vi "TimeTag_LSW_edits_Aug16.vi"() -> ()   [LabVIEW 2015]
doc: "This sample project is built upon the standard state machine template and shows how you could create an application that acquires, analyzes, and presents data. It includes functionality for presenting configuration dialogs, preserving settings between executions, loading and saving data, as well as exporting graph images and text files.\n\nIt is most appropriate for data that is acquired instantly as it does not allow for screen updates mid acquisition nor does it allow for continuous streaming to disk."
uses:
  <vilib>/ptbypt/NI_PtbyPt.lvlib
panel:
  out "Total Coin per sec":dbl
  out "Ch2/4 coin/sec":dbl(graph)
  out "Ch2/4 Total Coincidences":dbl
  out "Channel 2 CPS":dbl(graph)
  out "Channel 4 CPS":dbl(graph)
  out "Total Ch2 CPS":dbl
  out "Total Ch4 CPS":dbl
  in  "Averaging":dbl
  in  "Runs":dbl=100.0
  in  "Pulse TTL 2":bool
  in  "Pulse TTL 1":bool
  in  "Toggle\nTTL 2":bool
  in  "Toggle\nTTL 1":bool
  out "Total Starts":dbl
  in  "Record data":bool
  out "Initial time":dbl
  out "Elapsed time (s)":dbl
  out "FPGA_Run Status":dbl
  out "USB_Open Status":dbl
  out "Channel 4 Total\nCounts":dbl
  out "Channel 3 Total\nCounts":dbl
  out "Channel 2 Total\nCounts":dbl
  out "Channel 1 Total\nCounts":dbl
  in  "File Name":string="C:\\FPGA\\test.txt"
  out "?":dbl
  out "?":dbl
  out "?":dbl
  out "?":dbl
  out "stats":i64[](array[numeric])
  in  "Stop":bool
  out "Channel 4 CPS":dbl(knob) scale=0.0..2000000.0
  out "Channel 3 CPS":dbl(knob) scale=0.0..600.0
  out "Channel 2 CPS":dbl(knob) scale=0.0..700.0
  out "Channel 1 CPS":dbl(knob) scale=0.0..600.0
  # "Starts"
  # "Channel 1"
  # "Channel 2"
  # "Channel 3"
  # "Channel 4"
  # "Coincidence Channels 1 & 2"
  # "Coincidence Channels 1 & 3"
  # "Coincidence Channels 1 & 4"
  # "Coincidence Channels 2 & 3"
  # "Coincidence Channels 2 & 4"
  # "Coincidence Channels 3 & 4"
  # "Coincidence Channels 1 & 2 & 3"
  # "Coincidence Channels 1 & 2 & 4"
  # "Coincidence Channels 1 & 3 & 4"
  # "Coincidence Channels 2 & 3 & 4"
  # "Coincidence Channels 1 & 2 & 3 & 4"
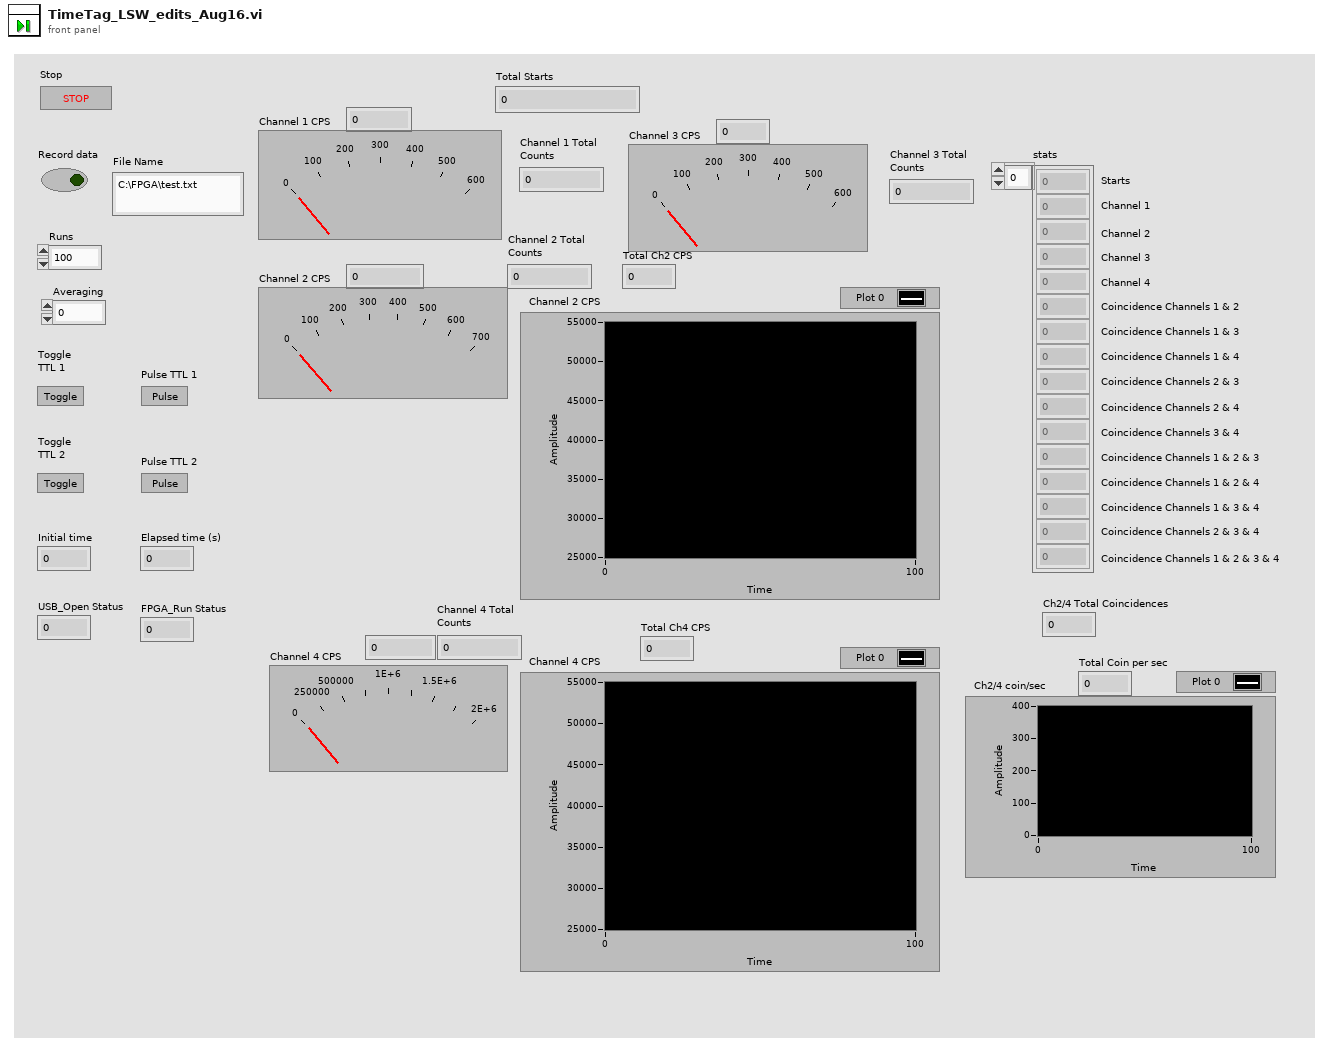
[diagram p1: front panel]
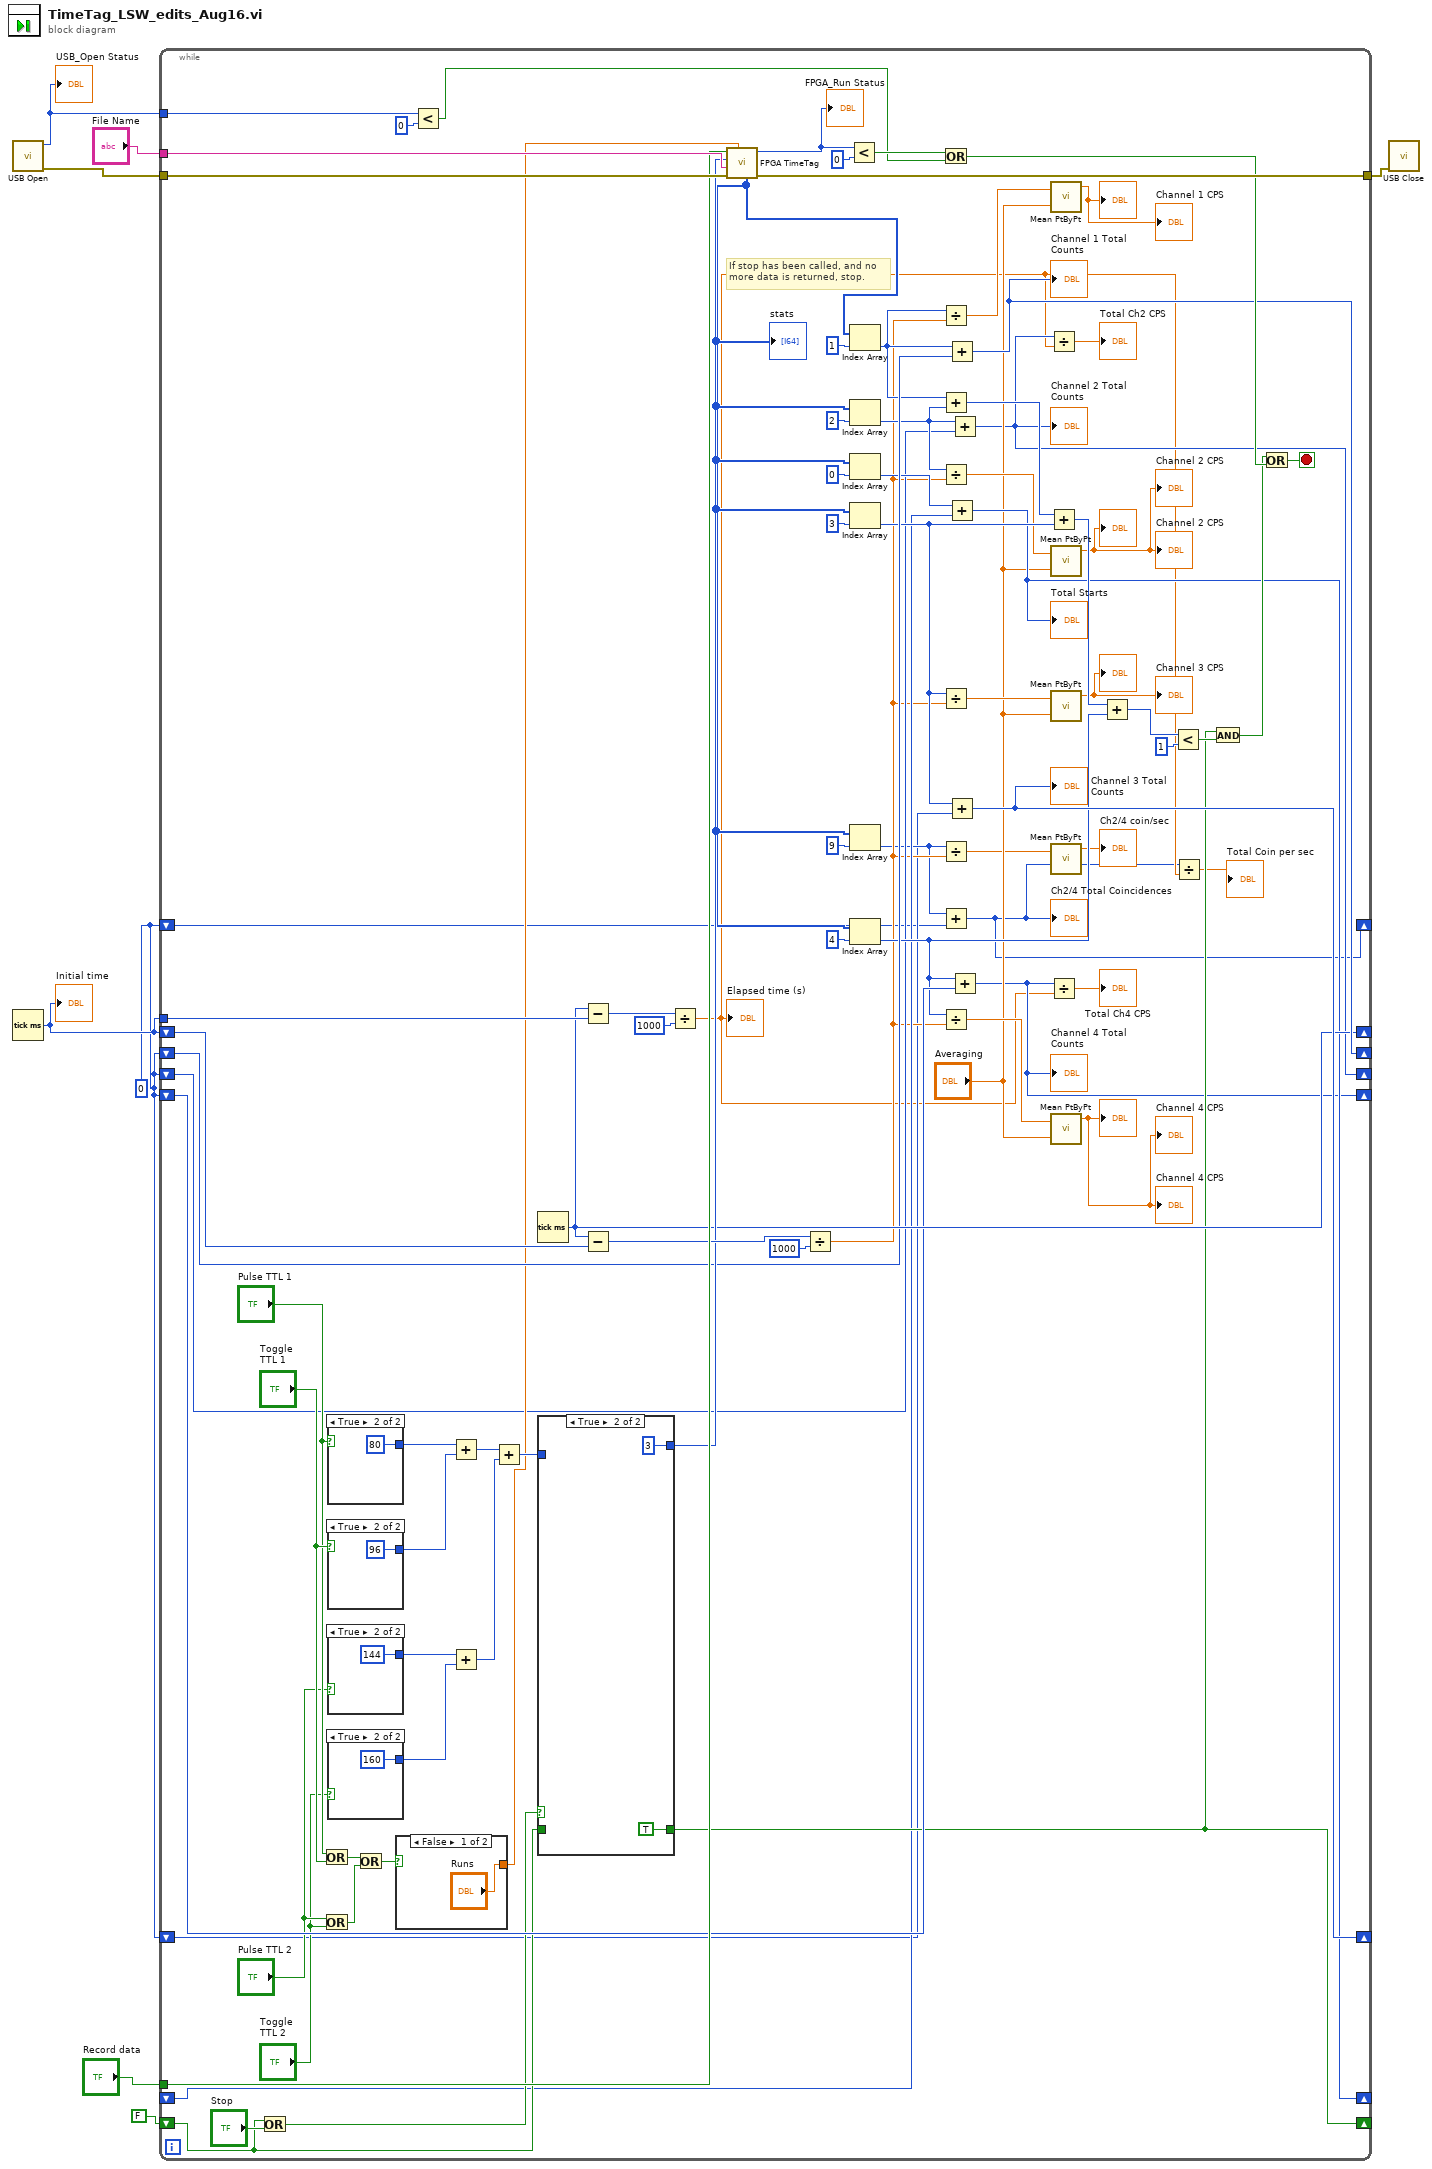
[diagram p0: block diagram]
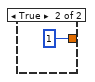
[diagram p2: hidden frame]
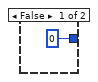
[diagram p3: hidden frame]
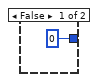
[diagram p4: hidden frame]
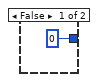
[diagram p5: hidden frame]
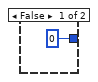
[diagram p6: hidden frame]
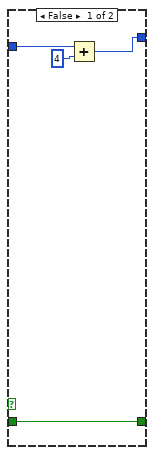
[diagram p7: hidden frame]
diagram:
  w1 = 0
  n1 = call "USB Open.vi"() -> ("error out"=w6:errorcluster, "function return"=w3:i32)  [unwired: 10 in]
  "USB_Open Status" <- w3
  n2 = Tick Count (ms)() -> (millisecond timer value=w4:u32)
  "Initial time" <- w4
  n3 = while {
    tunnel: w4 -> [w94]
    shift-right: [w72] -> _
    shift-left: w1 -> [w68]
    shift-right: [w24] -> _
    shift-left: w1 -> [w18]
    shift-right: [w71] -> _
    shift-left: w1 -> [w13]
    shift-right: [w25] -> _
    shift-left: w1 -> [w67]
    tunnel: w6 -> [w84]
    tunnel: [w85] -> w5
    tunnel: "Record data" -> [w82]
    tunnel: "File Name" -> [w83]
    shift-right: [w69] -> _
    shift-left: w4 -> [w80]
    tunnel: w3 -> [w76]
    shift-right: [w56] -> _
    shift-left: FALSE -> [w53]
    shift-right: [w49] -> _
    shift-left: _ -> [w50]
    shift-right: [w9] -> _
    shift-left: w1 -> [w12]
    stop <- w86 stop-if-true
    # "If stop has been called, and no\nmore data is returned, stop."
    n4 = Or(x=w53, y="Stop") -> (x .or. y?=w55:bool)
    n5 = Or(x="Pulse TTL 1", y="Toggle\nTTL 1") -> (x .or. y?=w40:bool)
    n6 = Or(x="Pulse TTL 2", y="Toggle\nTTL 2") -> (x .or. y?=w41:bool)
    n7 = case shown="True" "Pulse TTL 1" {
      tunnel: [0 80] -> w48
      frame False {
      }
      frame True {
      }
    }
    n8 = case shown="True" "Toggle\nTTL 1" {
      tunnel: [0 96] -> w47
      frame False {
      }
      frame True {
      }
    }
    n9 = case shown="True" "Pulse TTL 2" {
      tunnel: [0 144] -> w44
      frame False {
      }
      frame True {
      }
    }
    n10 = case shown="True" "Toggle\nTTL 2" {
      tunnel: [0 160] -> w45
      frame False {
      }
      frame True {
      }
    }
    n11 = Or(x=w40, y=w41) -> (x .or. y?=w42:bool)
    n12 = case shown="False" w42 {
      tunnel: ["Runs" 1] -> w38
      frame False {
      }
      frame True {
      }
    }
    n13 = Less?(x=w76, y=0) -> (x < y?=w74:bool)
    n14 = Add(x=w48, y=w47) -> (x+y=w46:i32)
    n15 = Add(x=w44, y=w45) -> (x+y=w43:i32)
    n16 = Add(x=w46, y=w43) -> (x+y=w39:i32)
    n17 = Tick Count (ms)() -> (millisecond timer value=w69:u32)
    n18 = case shown="True" w55 {
      tunnel: [w106 3] -> w70
      tunnel: [w108 TRUE] -> w56
      tunnel: w53 -> [w108 _]
      tunnel: w39 -> [w105 _]
      frame False {
        n19 = Add(x=w105, y=4) -> (x+y=w106:i32)
      }
      frame True {
      }
    }
    n20 = Subtract(x=w69, y=w94) -> (x-y=w93:u32)
    n21 = Subtract(x=w69, y=w80) -> (x-y=w79:u32)
    n22 = Divide(x=w93, y=1000) -> (x/y=w10:dbl)
    "Elapsed time (s)" <- w10
    n23 = call "FPGA TimeTag.vi"("runs"=w38, "error in (no error)"=w84, "fileName"=w83, "fpgaCommand"=w70, "saveData"=w82) -> ("error out"=w85:errorcluster, "function return"=w81:i32, "stats"=w20:i64[])  [unwired: 4 in]
    "stats" <- w20
    "FPGA_Run Status" <- w81
    n24 = Divide(x=w79, y=1000) -> (x/y=w17:dbl)
    n25 = Less?(x=w81, y=0) -> (x < y?=w75:bool)
    n26 = Index Array(array=w20, index=1) -> (element=w59:i64)
    n27 = Index Array(array=w20, index=2) -> (element=w66:i64)
    n28 = Index Array(array=w20, index=0) -> (element=w51:i64)
    n29 = Index Array(array=w20, index=3) -> (element=w62:i64)
    n30 = Index Array(array=w20, index=9) -> (element=w14:i64)
    n31 = Index Array(array=w20, index=4) -> (element=w63:i64)
    n32 = Or(x=w75, y=w74) -> (x .or. y?=w73:bool)
    n33 = Divide(x=w59, y=w17) -> (x/y=w33:dbl)
    n34 = Add(x=w59, y=w66) -> (x+y=w61:i64)
    n35 = Divide(x=w66, y=w17) -> (x/y=w32:dbl)
    n36 = Divide(x=w62, y=w17) -> (x/y=w31:dbl)
    n37 = Divide(x=w14, y=w17) -> (x/y=w16:dbl)
    n38 = Add(x=w14, y=w12) -> (x+y=w9:i64)
    "Ch2/4 Total Coincidences" <- w9
    n39 = Divide(x=w63, y=w17) -> (x/y=w29:dbl)
    n40 = Add(x=w59, y=w68) -> (x+y=w72:i64)
    "Channel 1 Total\nCounts" <- w72
    n41 = Add(x=w51, y=w50) -> (x+y=w49:i64)
    "Total Starts" <- w49
    n42 = Add(x=w62, y=w13) -> (x+y=w71:i64)
    "Channel 3 Total\nCounts" <- w71
    n43 = Add(x=w66, y=w18) -> (x+y=w24:i64)
    "Channel 2 Total\nCounts" <- w24
    n44 = Add(x=w63, y=w67) -> (x+y=w25:i64)
    "Channel 4 Total\nCounts" <- w25
    n45 = Divide(x=w24, y=w10) -> (x/y=→"Total Ch2 CPS":dbl)
    n46 = Add(x=w61, y=w62) -> (x+y=w65:i64)
    n47 = Divide(x=w25, y=w10) -> (x/y=→"Total Ch4 CPS":dbl)
    n48 = call <vilib>:"Mean PtByPt.vi"("x"=w33, "sample length"="Averaging") -> ("mean"=→"Channel 1 CPS" →"?":dbl)  [unwired: 2 in, 1 out]
    n49 = call <vilib>:"Mean PtByPt.vi"("x"=w32, "sample length"="Averaging") -> ("mean"=→"Channel 2 CPS" →"?" →"Channel 2 CPS":dbl)  [unwired: 2 in, 1 out]
    n50 = call <vilib>:"Mean PtByPt.vi"("x"=w31, "sample length"="Averaging") -> ("mean"=→"Channel 3 CPS" →"?":dbl)  [unwired: 2 in, 1 out]
    n51 = call <vilib>:"Mean PtByPt.vi"("x"=w16) -> ("mean"=→"Ch2/4 coin/sec":dbl)  [unwired: 3 in, 1 out]
    n52 = call <vilib>:"Mean PtByPt.vi"("x"=w29, "sample length"="Averaging") -> ("mean"=→"Channel 4 CPS" →"?" →"Channel 4 CPS":dbl)  [unwired: 2 in, 1 out]
    n53 = Add(x=w65, y=w63) -> (x+y=w64:i64)
    n54 = Less?(x=w64, y=1) -> (x < y?=w58:bool)
    n55 = Divide(x=w9, y=w10) -> (x/y=→"Total Coin per sec":dbl)
    n56 = And(x=w56, y=w58) -> (x .and. y?=w57:bool)
    n57 = Or(x=w57, y=w73) -> (x .or. y?=w86:bool)
  }
  n58 = call "USB Close.vi"("error in (no error)"=w5) -> ()  [unwired: 9 in, 2 out]
